vi "Main.vi"() -> ()   [LabVIEW 2017]
doc: "This template is for the Queued Message Handler design pattern.\n\nThe Event Handling Loop generates messages based on user interface actions.\n\nThe Message Handling Loop processes messages generated by the Event Handling Loop, or by other messages. The messages are string values, so new messages can be added easily to the Message Cases case structure in the Message Handling Loop. Each message cluster can also provide an optional value for Message Data, which is a variant that can be converted to whatever message-specific data is required."
uses:
  Controls/Main Tabs.ctl
  Controls/Auto.ctl
  Controls/UI Data.ctl
  support/Message Queue/Enqueue Message (Single).vi
  <vilib>/Utility/error.llb/Error Cluster From Error Code.vi
  <vilib>/ErrorRing/Error Ring.xnode
  support/Message Queue/Message Queue.lvlib
  support/User Event - Stop/User Event - Stop.lvlib
panel:
  out "Date-Time":string
  out "Main Tab":T1
  in  "Autocycle":T2
  in  "Manual":bool
  in  "Parameters":bool
  in  "Maintenance":bool
  in  "Save Para":bool
  in  "Home Para":bool
  in  "ParaTab":T3(tab)
  in  "StopperRearDelay":dbl format="%#.2f"
  in  "StopperFrontDelay":dbl format="%#.2f"
  in  "MaxAlarms":dbl caption="Max Alarms in 1 Minute" format="%#.2f"
  in  "MaxConsecutive":dbl caption="Max Consecutive Alarms" format="%#.2f"
  in  "Gate Close Delay":dbl format="%#.2f"
  in  "Gate Open Delay":dbl format="%#.2f"
  in  "BF Off Delay":dbl format="%#.2f"
  in  "BF On Delay":dbl format="%#.2f"
  in  "DelayAfterReject":dbl format="%#.2f"
  in  "MeasurementTime":dbl format="%#.2f"
  in  "DelayAfterMesFront":dbl format="%#.2f"
  in  "DelayAfterCut":dbl format="%#.2f"
  in  "DelayAfterCutClamp":dbl format="%#.2f"
  in  "DelayAfterInsClamp":dbl format="%#.2f"
  in  "DelayToClose":dbl format="%#.2f"
  in  "DelayToOpen":dbl format="%#.2f"
  in  "DelayAfterInsertion":dbl format="%#.2f"
  in  "DelayBeforeInsertion":dbl format="%#.2f"
  in  "AgitatorUpTime":dbl format="%#.2f"
  in  "AgitatorDownTime":dbl format="%#.2f"
  in  "All IO":bool
  in  "Stats":bool
  in  "Home AC":bool
  out "Status":string
  out "Count":dbl format="%06.0f"
  out "Count 3":dbl caption="Cycle Time" format="%0.2f"
  out "Count 2":dbl caption="Rejects" format="%06.0f"
  in  "Statuses":string[][](table)
  in  "Exit":bool
  # "Dip-Tube Assembly Automation"
  # "Vision Harmony Dip-Tube Assembly Automation"
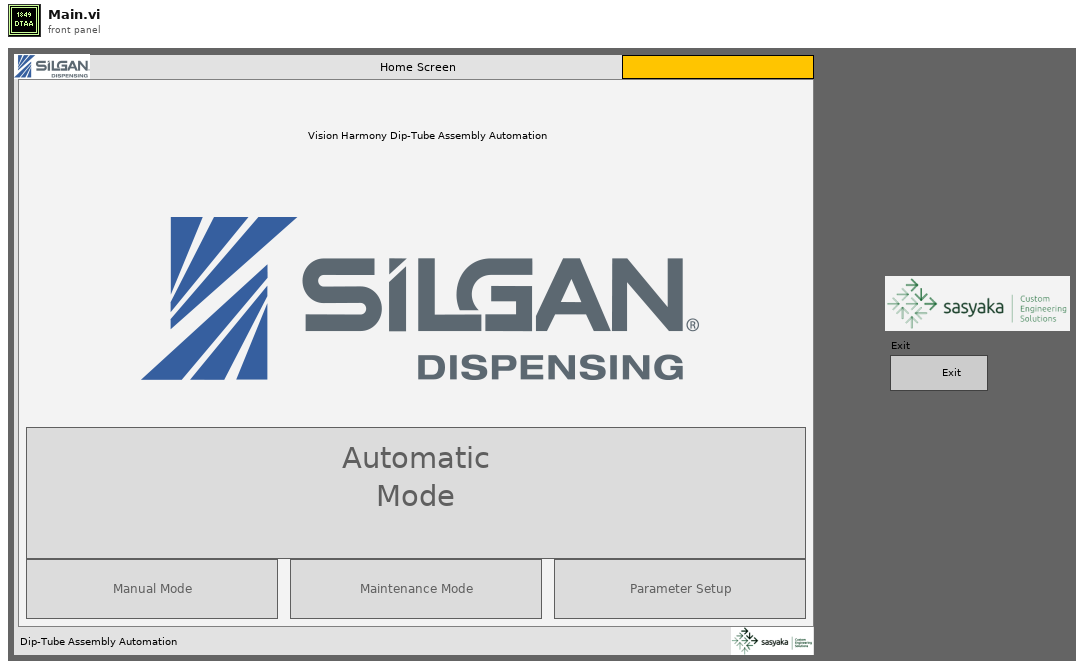
[diagram p1: front panel]
types:
  T1 = typedef "Main Tabs.ctl" = enum32{"Home Screen", "Parameter Setup", "Manual Mode", "Autocycle"}
  T2 = typedef "Auto.ctl" = bool
  T3 = enum32{"General & Indexing", "Bowl Feeder & Pump Conveyor", "Cutting, Measurement & Rejection", "Tube Feeder & Insertion"}
  T4 = typedef "UI Data.ctl" = cluster{"Main Tab":refnum<vi>}
  T5 = typedef "Message Queue.lvlib/All Message Queues.ctl" = cluster{"UI":refnum<queue>}
  T6 = enum8{"Enabled", "Disabled", "Disabled and Grayed Out"}
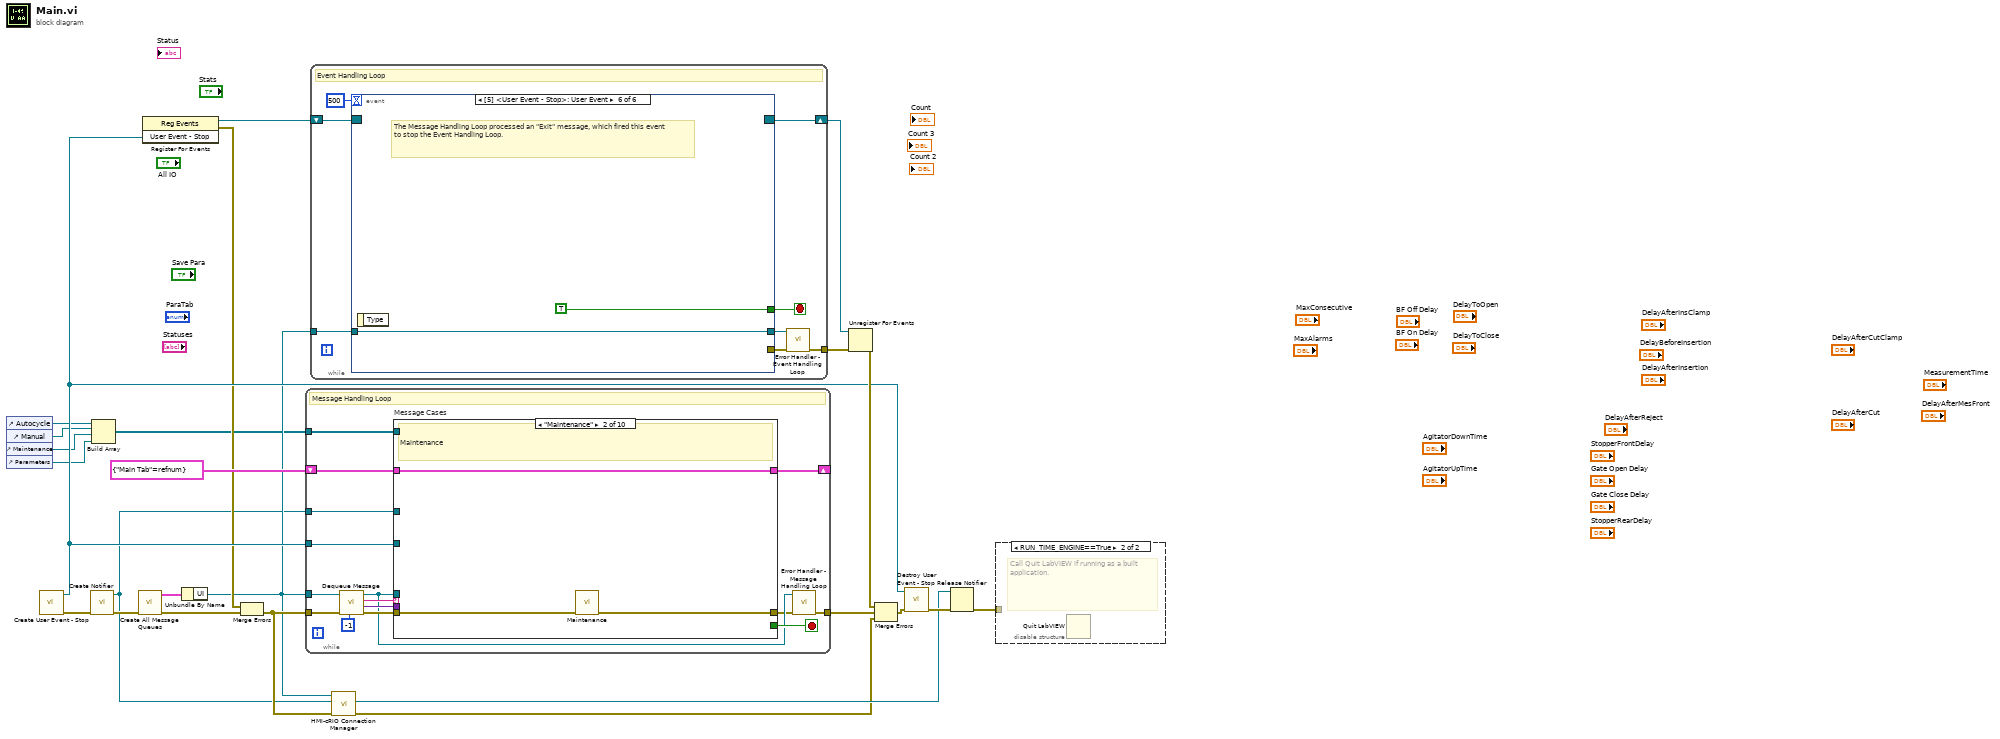
[diagram p0: block diagram]
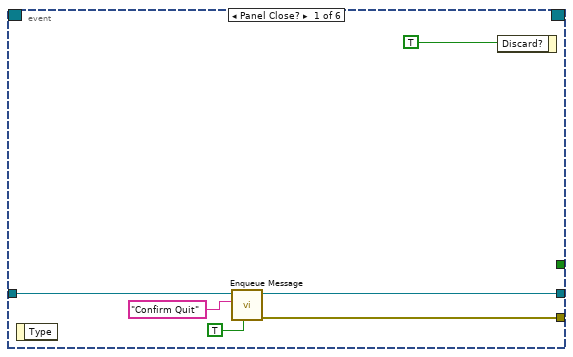
[diagram p2: hidden frame]
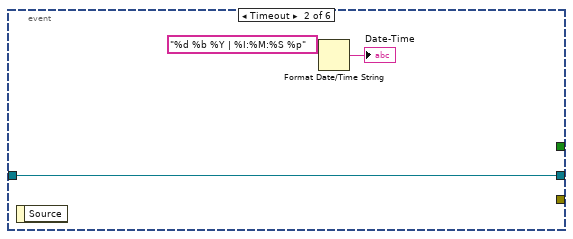
[diagram p3: hidden frame]
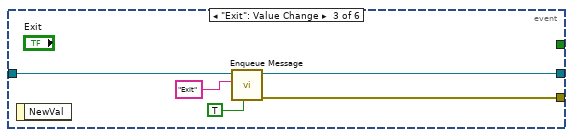
[diagram p4: hidden frame]
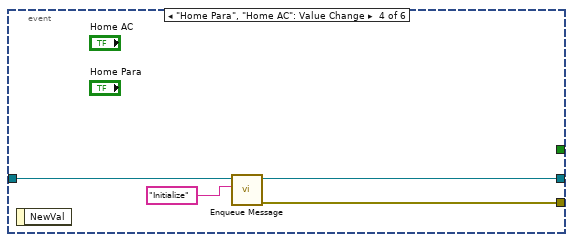
[diagram p5: hidden frame]
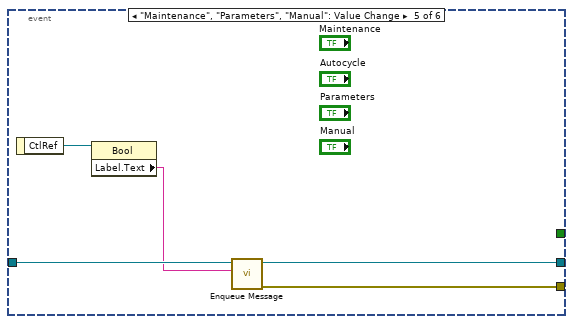
[diagram p6: hidden frame]
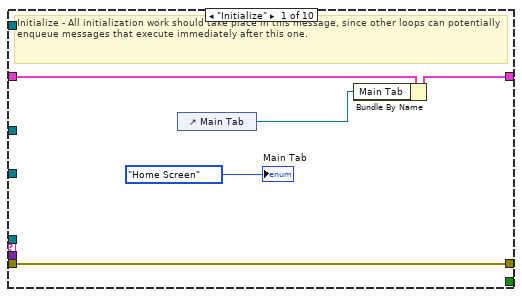
[diagram p7: hidden frame]
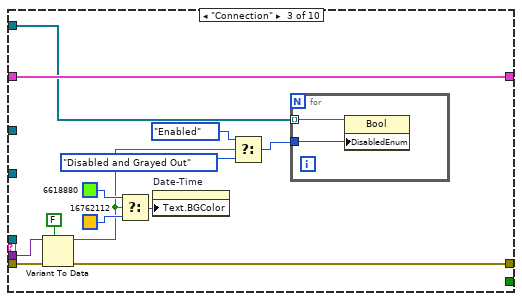
[diagram p8: hidden frame]
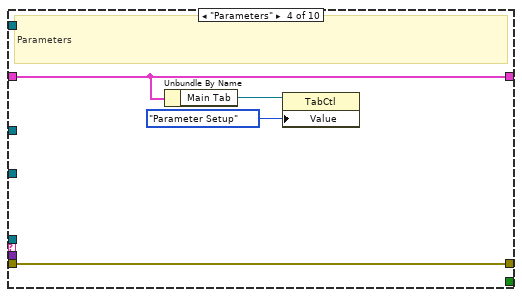
[diagram p9: hidden frame]
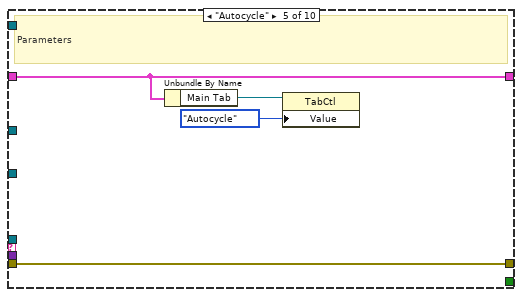
[diagram p10: hidden frame]
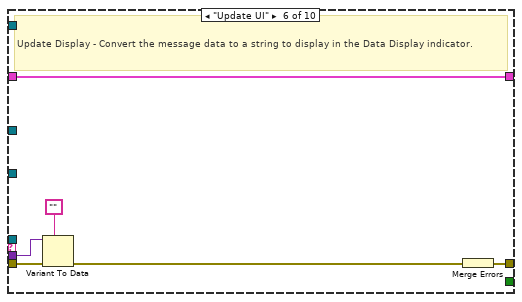
[diagram p11: hidden frame]
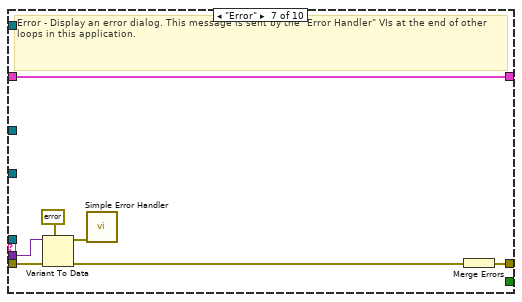
[diagram p12: hidden frame]
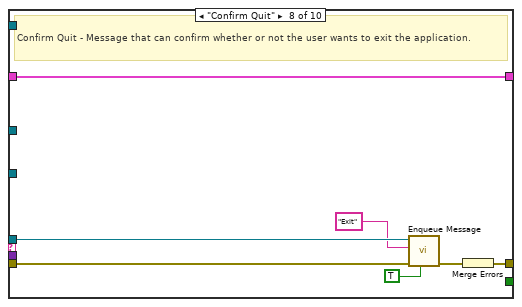
[diagram p13: hidden frame]
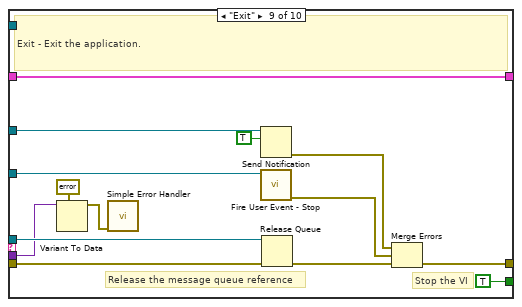
[diagram p14: hidden frame]
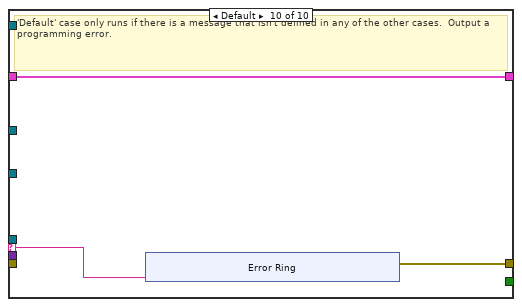
[diagram p15: hidden frame]
diagram:
  n1 = control-ref of="Autocycle"() -> (w5:refnum<vi>)
  n2 = control-ref of="Manual"() -> (w4:refnum<vi>)
  n3 = control-ref of="Maintenance"() -> (w3:refnum<vi>)
  n4 = control-ref of="Parameters"() -> (w2:refnum<vi>)
  n5 = call "Create User Event - Stop.vi"() -> ("error out"=w12:errorcluster, "User Event - Stop"=w16:refnum<user-event>)  [unwired: 10 in]
  n6 = call "Create Notifier.vi"("error in (no error)"=w12) -> ("error out"=w11:errorcluster, "notifier out"=w6:refnum<notifier>)  [unwired: 9 in]
  n7 = Build Array(w5, w4, w3, w2) -> (w1:refnum<vi>[])
  n8 = call "Create All Message Queues.vi"("error in (no error)"=w11) -> ("error out"=w25:errorcluster, "Message Queues out"=w24:T5)  [unwired: 9 in]
  n9 = register-events(w16) -> (reference out=w17:refnum<event-registration>, error out=w15:errorcluster)  [unwired: 2 in]
  n10 = Unbundle By Name(w24) -> ("UI"=w13:refnum<queue>)
  n11 = Merge Errors(w15, w25) -> (w14:errorcluster)
  n12 = while {
    tunnel: w13 -> [w32]
    shift-right: [w39] -> _
    shift-left: T4 {"Main Tab"=refnum} ("Data Cluster") -> [w40]
    tunnel: w16 -> [w37]
    tunnel: w14 -> [w36]
    tunnel: [w30] -> w23
    tunnel: w6 -> [w27]
    tunnel: w1 -> [w26]
    stop <- w38 stop-if-true
    # "Message Handling Loop"
    n13 = call "Dequeue Message.vi"("timeout"=-1, "error in (no error)"=w36, "Message Queue"=w32) -> ("error out"=w35:errorcluster, "Message Data"=w33:variant, "Message"=w34:string, "dup Message Queue"=w31:refnum<queue>)  [unwired: 5 in]
    n14 = case "Message Cases" shown="\"Maintenance\"" w34 {
      selector: w34 -> [_ _ _ _ _ _ _ _ _ w106]
      tunnel: w31 -> [_ _ _ _ _ _ _ w87 w105 _]
      tunnel: w35 -> [w45 w47 w59 w67 w71 w75 w84 w91 w98 _]
      tunnel: [w45 w46 w58 w67 w71 w76 w78 w89 w101 w107] -> w29
      tunnel: w40 -> [w44 w48 w61 w66 w70 w77 w83 w90 w104 w108]
      tunnel: [w43 w48 w61 w66 w70 w77 w83 w90 w104 w108] -> w39
      tunnel: [_ _ _ _ _ _ _ _ TRUE _] -> w38
      tunnel: w33 -> [_ _ w57 _ _ w74 w82 _ w95 _]
      tunnel: w37 -> [_ _ _ _ _ _ _ _ w100 _]
      tunnel: w27 -> [_ _ _ _ _ _ _ _ w94 _]
      tunnel: w26 -> [_ _ w53 _ _ _ _ _ _ _]
      frame "Initialize" {
        # "Initialize - All initialization work should take place in this message, since other loops can potentially enqueue messages that execute immediately after this one."
        n15 = control-ref of="Main Tab"() -> (w42:refnum<vi>)
        n16 = Bundle By Name(cluster=w44, "Main Tab"=w42) -> (w43:T4)
        "Main Tab" <- Main_Tabs."Home Screen" ("Main Tab")
      }
      frame "Maintenance" {
        # "Maintenance"
        n17 = call "Maintenance.vi"("Error In"=w47) -> ("Error out"=w46:errorcluster)  [unwired: 10 in]
      }
      frame "Connection" {
        n18 = Variant To Data(error in=w59, type=FALSE, Variant=w57) -> (data=w52:bool, error out=w58:errorcluster)
        n19 = Select(t=u32 6618880 ("Text.Text Colors:BG Color"), s=w52, f=u32 16762112 ("Text.Text Colors:BG Color")) -> (s? t:f=w54:u32)
        n20 = property on="Date-Time" class="Str"("Text.BGColor"=w54) -> ()  [unwired: 2 in, 2 out]
        n21 = Select(t=T6."Enabled" ("Disabled"), s=w52, f=T6."Disabled and Grayed Out") -> (s? t:f=w50:T6)
        n22 = for {
          tunnel: w53 -> [w63] mode=indexing
          tunnel: w50 -> [w62]
          n23 = property class="Bool"(reference=w63, "DisabledEnum"=w62) -> ()  [unwired: 1 in, 2 out]
        }
      }
      frame "Parameters" {
        # "Parameters"
        n24 = Unbundle By Name(w66) -> ("Main Tab"=w65:refnum<vi>)
        n25 = property class="TabCtl"(reference=w65, "Value"=Main_Tabs."Parameter Setup" ("Main Tab")) -> ()  [unwired: 1 in, 2 out]
      }
      frame "Autocycle" {
        # "Parameters"
        n26 = Unbundle By Name(w70) -> ("Main Tab"=w69:refnum<vi>)
        n27 = property class="TabCtl"(reference=w69, "Value"=Main_Tabs."Autocycle" ("Main Tab")) -> ()  [unwired: 1 in, 2 out]
      }
      frame "Update UI" {
        # "Update Display - Convert the message data to a string to display in the Data Display indicator."
        n28 = Variant To Data(error in=w75, type="", Variant=w74) -> (error out=w72:errorcluster)  [unwired: 1 out]
        n29 = Merge Errors(w72) -> (w76:errorcluster)
      }
      frame "Error" {
        # "Error - Display an error dialog. This message is sent by the \"Error Handler\" VIs at the end of other loops in this application."
        n30 = Variant To Data(error in=w84, type=errorcluster {"status"=FALSE, "code"=0, "source"=""} ("error constant"), Variant=w82) -> (data=w80:errorcluster, error out=w79:errorcluster)
        n31 = call <vilib>:"Simple Error Handler.vi"("error in (no error)"=w80) -> ()  [unwired: 4 in, 5 out]
        n32 = Merge Errors(w79) -> (w78:errorcluster)
      }
      frame "Confirm Quit" {
        # "Confirm Quit - Message that can confirm whether or not the user wants to exit the application."
        n33 = call-poly "Enqueue Message.vi"("Priority Message? (F)"=TRUE, "error in (no error)"=w91, "Message"="Exit", "Message Queue"=w87) -> ("error out"=w88:errorcluster)  [unwired: 6 in, 1 out]
        n34 = Merge Errors(w88) -> (w89:errorcluster)
      }
      frame "Exit" {
        # "Stop the VI"
        # "Release the message queue reference"
        # "Exit - Exit the application."
        n35 = Variant To Data(type=errorcluster {"status"=FALSE, "code"=0, "source"=""} ("error constant"), Variant=w95) -> (data=w96:errorcluster)  [unwired: 1 in, 1 out]
        n36 = call <vilib>:"Simple Error Handler.vi"("error in (no error)"=w96) -> ()  [unwired: 4 in, 5 out]
        n37 = Send Notification(notification=TRUE, notifier=w94) -> (error out=w92:errorcluster)  [unwired: 1 in, 1 out]
        n38 = call "Fire User Event - Stop.vi"("User Event - Stop"=w100) -> ("error out"=w99:errorcluster)  [unwired: 10 in]
        n39 = Release Queue(queue=w105, error in (no error)=w98) -> (error out=w102:errorcluster)  [unwired: 1 in, 2 out]
        n40 = Merge Errors(w92, w99, w102) -> (w101:errorcluster)
      }
      frame Default {
        # "'Default' case only runs if there is a message that isn't defined in any of the other cases.  Output a programming error."
        n41 = xnode "Error Ring"("parameter 0"=w106) -> ("error out"=w107:errorcluster)
      }
    }
    n42 = call "Error Handler - Message Handling Loop.vi"("error in (no error)"=w29, "Message Queue"=w31) -> ("dup error in"=w30:errorcluster)  [unwired: 8 in, 1 out]
  }
  n43 = while {
    tunnel: w13 -> [w123]
    shift-right: [w121] -> w20
    shift-left: w17 -> [w122]
    tunnel: [w117] -> w18
    stop <- w119 stop-if-true
    # "Event Handling Loop"
    n44 = event shown="[5] <User Event - Stop>: User Event" {
      selector: w122 -> [_ _ _ _ _ _]
      dyn-events: [_ _ _ _ _ _] -> w121
      timeout: 500 -> [_ _ _ _ _ _]
      tunnel: [_ _ _ _ _ TRUE ("Discard?")] -> w119
      tunnel: w123 -> [w128 w132 w137 w141 w146 w148]
      tunnel: [w127 _ w136 w140 w145 _] -> w120
      tunnel: [w126 w132 w135 w139 w144 w148] -> w118
      event Panel Close? {
        n45 = event-data() -> ()  [unwired: 1 in, 1 out]
        n46 = call-poly "Enqueue Message.vi"("Priority Message? (F)"=TRUE, "Message"="Confirm Quit", "Message Queue"=w128) -> ("error out"=w127:errorcluster, "dup Message Queue"=w126:refnum<queue>)  [unwired: 7 in]
        n47 = event-data("Discard?"=TRUE) -> ()  [unwired: 1 in, 1 out]
      }
      event Timeout {
        n48 = event-data() -> ()  [unwired: 1 in, 1 out]
        n49 = Format Date/Time String(time format string (%c)="%d %b %Y | %I:%M:%S %p") -> (date/time string=→"Date-Time":string)  [unwired: 2 in]
      }
      event "Exit": Value Change {
        n50 = event-data() -> ()  [unwired: 1 in, 1 out]
        n51 = call-poly "Enqueue Message.vi"("Priority Message? (F)"=TRUE, "Message"="Exit", "Message Queue"=w137) -> ("error out"=w136:errorcluster, "dup Message Queue"=w135:refnum<queue>)  [unwired: 7 in]
      }
      event "Home Para", "Home AC": Value Change {
        n52 = event-data() -> ()  [unwired: 1 in, 1 out]
        n53 = call-poly "Enqueue Message.vi"("Message"="Initialize", "Message Queue"=w141) -> ("error out"=w140:errorcluster, "dup Message Queue"=w139:refnum<queue>)  [unwired: 8 in]
      }
      event "Maintenance", "Parameters", "Manual": Value Change {
        n54 = event-data() -> ("CtlRef"=w143:refnum<vi>)  [unwired: 1 in]
        n55 = property class="Bool"(reference=w143) -> ("Label.Text"=w142:string)  [unwired: 1 in, 2 out]
        n56 = call-poly "Enqueue Message.vi"("Message"=w142, "Message Queue"=w146) -> ("error out"=w145:errorcluster, "dup Message Queue"=w144:refnum<queue>)  [unwired: 8 in]
      }
      event User Event {
        # "The Message Handling Loop processed an \"Exit\" message, which fired this event to stop the Event Handling Loop."
        n57 = event-data() -> ()  [unwired: 1 in, 1 out]
      }
    }
    n58 = call "Error Handler - Event Handling Loop.vi"("error in (no error)"=w120, "Message Queue"=w118) -> ("dup error in"=w117:errorcluster)  [unwired: 8 in, 1 out]
  }
  n59 = call "HMI-cRIO Connection Manager.vi"("error in"=w14, "notifier in"=w6, "Queue in"=w13) -> ("error out"=w7:errorcluster, "Notifier out"=w8:refnum<notifier>)  [unwired: 7 in]
  n60 = Unregister For Events(event registration refnum=w20, error in=w18) -> (error out=w21:errorcluster)
  n61 = Merge Errors(w21, w23, w7) -> (w22:errorcluster)
  n62 = call "Destroy User Event - Stop.vi"("error in (no error)"=w22, "User Event - Stop"=w16) -> ("error out"=w10:errorcluster)  [unwired: 9 in]
  n63 = Release Notifier(notifier=w8, error in (no error)=w10) -> (error out=w9:errorcluster)  [unwired: 1 in, 2 out]
  n64 = disable-structure shown="RUN_TIME_ENGINE==True" {
    disable-tunnel: w9 -> [_ _]
    frame condition #0 (active) {
    }
    frame condition #1 {
      # "Call Quit LabVIEW if running as a built application."
      n65 = Quit LabVIEW() -> ()  [unwired: 1 in]
    }
  }
